vi "Comment parser.vi"   [LabVIEW 2015]
doc: "This polymorphic VI parsed out the \"comments\"\nIn text based programming language uses different ways to comment code lines\nThis Polymorphc VI contains:\n\nThe C/C++ comment convention\n// comment line\n/* comment block */\n\nThe Python comment convention\n# comment line"
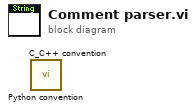
[diagram p0: block diagram]
diagram:
  n1 = call "Python convention.vi"() -> ()  [unwired: 26 in, 2 out]
  n2 = call "C_C++ convention.vi"() -> ()  [unwired: 26 in, 2 out]
